vi "save position data.vi"(10 "step name":string, 11 "Motion.lvclass":refnum<class "Motion.lvclass">) -> (3 "Motion.lvclass 2":refnum<class "Motion.lvclass">)   [LabVIEW 2016]
uses:
  Classes/Controller/Motion/Motion.lvclass
panel:
  out "appended path":path
  out "concatenated string":string
  out "spreadsheet string":string
  in  "Array":dbl[](array[numeric])
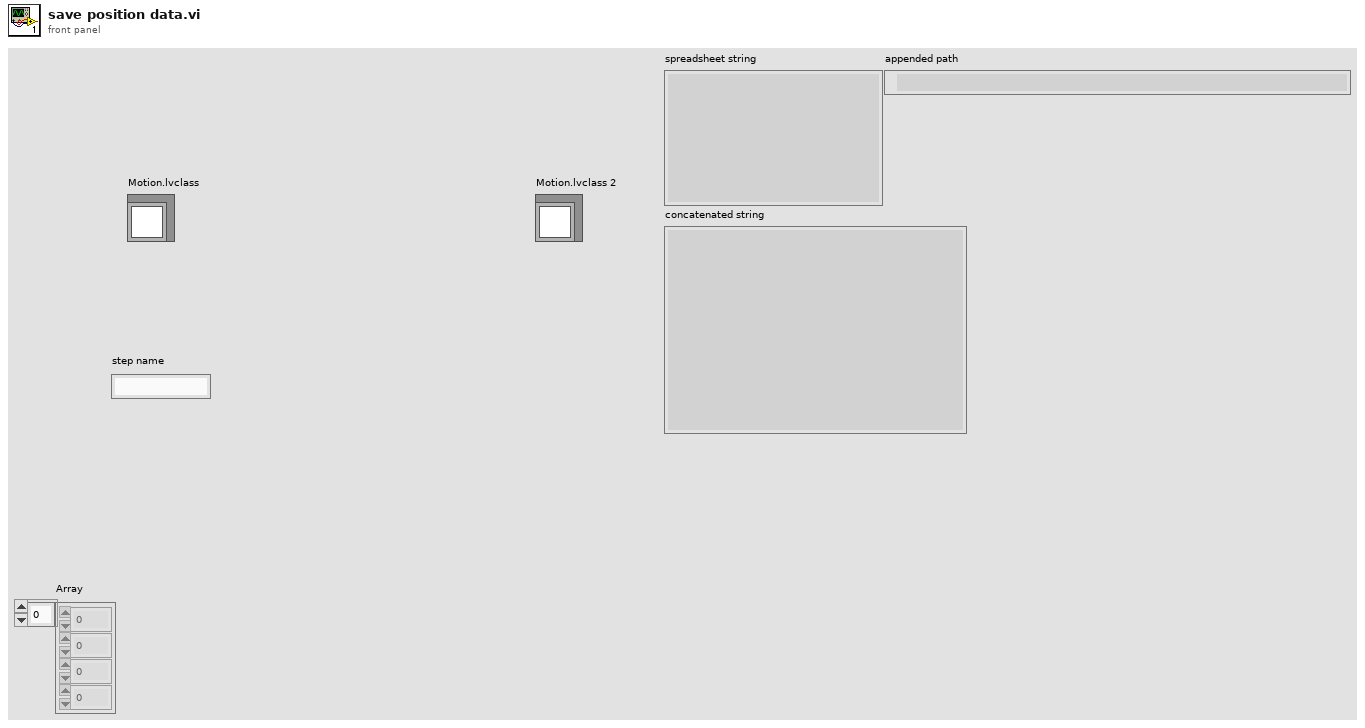
[diagram p1: front panel]
types:
  T1 = enum16{"open", "replace", "create", "open or create", "replace or create", "replace or create with confirmation"}
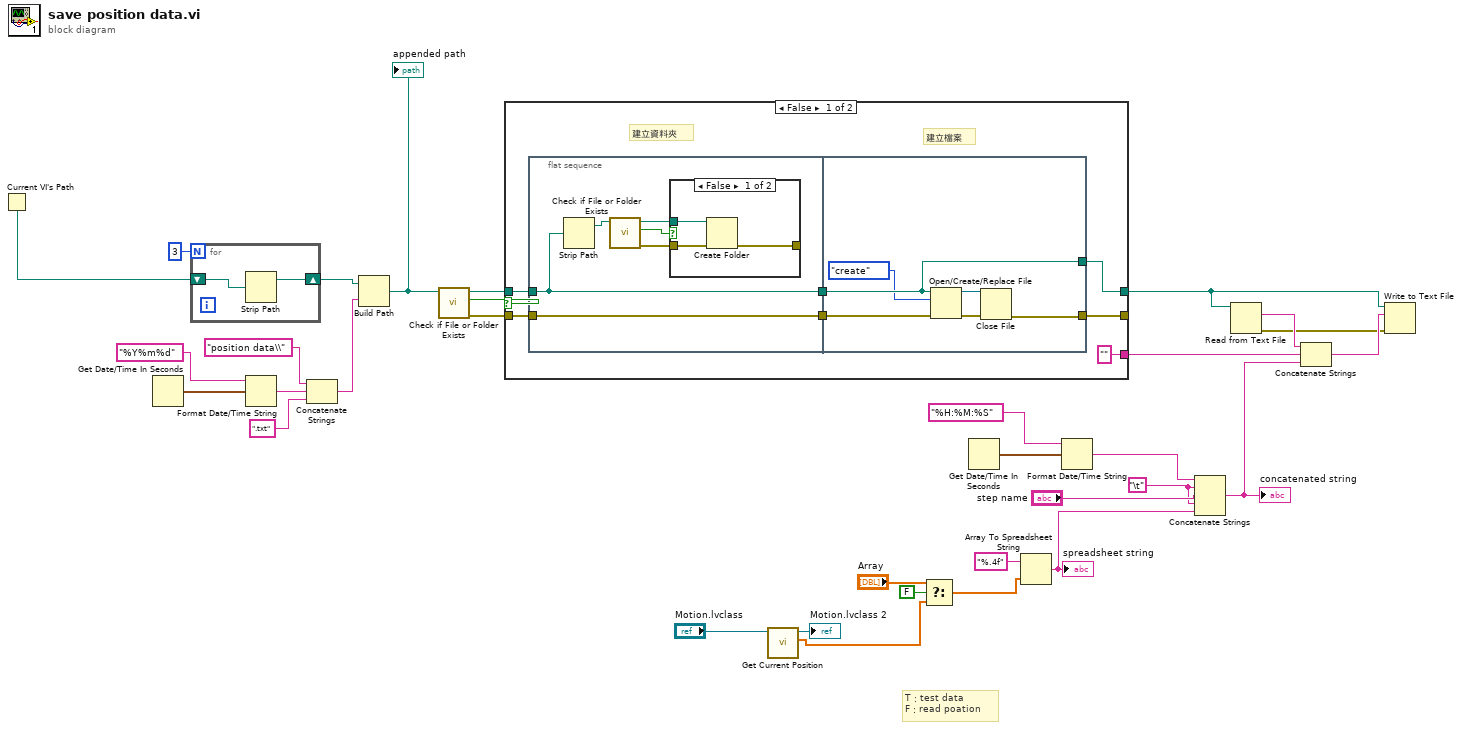
[diagram p0: block diagram]
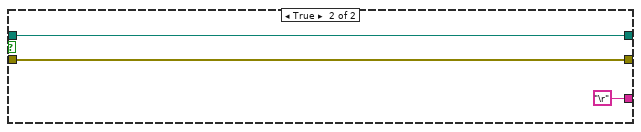
[diagram p3: hidden frame]
diagram:
  w26 = "\t"
  # "T：test data\nF：read poation"
  n1 = Current VI's Path() -> (path=w18:path)
  n2 = Get Date/Time In Seconds() -> (seconds since 1Jan1904=w22:timestamp)
  n3 = for {
    N: 3 -> [_]
    shift-right: [w34] -> w19
    shift-left: w18 -> [w33]
    n4 = Strip Path(path=w33) -> (stripped path=w34:path)  [unwired: 1 out]
  }
  n5 = Format Date/Time String(time format string (%c)="%Y%m%d", seconds (now)=w22) -> (date/time string=w16:string)  [unwired: 1 in]
  n6 = Concatenate Strings("position data\\" ("string"), w16, ".txt" ("string")) -> (w17:string)
  n7 = Build Path(base path=w19, name or relative path=w17) -> (appended path=w20:path)
  "appended path" <- w20
  n8 = call <vilib>:"Check if File or Folder Exists.vi"("path"=w20) -> ("error out"=w23:errorcluster, "file or folder exists?"=w25:bool, "dup path"=w24:path)  [unwired: 8 in]
  n9 = case shown="False" w25 {
    tunnel: w24 -> [w40 w60]
    tunnel: w23 -> [w41 w59]
    tunnel: [w39 w59] -> _
    tunnel: [w38 w60] -> w8
    tunnel: ["" "\r"] -> w7
    frame False {
      # "建立檔案"
      # "建立資料夾"
      n10 = flat-sequence {
        tunnel: w40 -> [w42]
        tunnel: w41 -> [w47]
        tunnel: [w47] -> w37
        tunnel: [w42] -> w36
        tunnel: [w52] -> w39
        tunnel: [w56] -> w38
        tunnel: w37 -> [w57]
        tunnel: w36 -> [w56]
        frame #0 {
          n11 = Strip Path(path=w42) -> (stripped path=w43:path)  [unwired: 1 out]
          n12 = call <vilib>:"Check if File or Folder Exists.vi"("path"=w43) -> ("error out"=w46:errorcluster, "file or folder exists?"=w44:bool, "dup path"=w45:path)  [unwired: 8 in]
          n13 = case shown="False" w44 {
            tunnel: w45 -> [w50 _]
            tunnel: [w49 w51] -> _
            tunnel: w46 -> [w48 w51]
            frame False {
              n14 = Create Folder(path (use dialog)=w50, error in=w48) -> (error out=w49:errorcluster)  [unwired: 1 in, 2 out]
            }
            frame True {
            }
          }
        }
        frame #1 {
          n15 = Open/Create/Replace File(file path (use dialog)=w56, error in=w57, operation (0:open)=T1."create") -> (refnum out=w54:refnum<file>, error out=w53:errorcluster)  [unwired: 3 in, 1 out]
          n16 = Close File(refnum=w54, error in=w53) -> (error out=w52:errorcluster)  [unwired: 1 out]
        }
      }
    }
    frame True {
    }
  }
  n17 = call-dynamic "Get Current Position.vi"("Motion in"="Motion.lvclass") -> ("XYZTheta Out"=w1:dbl[], "Motion out"=→"Motion.lvclass 2":refnum<class "Motion.lvclass">)  [unwired: 8 in, 1 out]
  n18 = Select(t="Array", s=FALSE, f=w1) -> (s? t:f=w4:dbl[])
  n19 = Get Date/Time In Seconds() -> (seconds since 1Jan1904=w31:timestamp)
  n20 = Array To Spreadsheet String(array=w4, 3:"%.4f" ("format string")) -> (spreadsheet string=w28:string)  [unwired: 1 in]
  "spreadsheet string" <- w28
  n21 = Format Date/Time String(time format string (%c)="%H:%M:%S", seconds (now)=w31) -> (date/time string=w29:string)  [unwired: 1 in]
  n22 = Concatenate Strings(w29, w26, "step name", w26, w28) -> (w9:string)
  "concatenated string" <- w9
  n23 = Read from Text File(file (use dialog)=w8) -> (text=w12:string, error out=w10:errorcluster)  [unwired: 3 in, 2 out]
  n24 = Concatenate Strings(w12, w7, w9) -> (w11:string)
  n25 = Write to Text File(file (use dialog)=w8, text=w11, error in=w10) -> ()  [unwired: 1 in, 3 out]
